vi "PulseHistogram.vi"() -> ()   [LabVIEW 2012]
doc: "This example demonstrates how to generate and acquire data up to eight channels using an NI 6587 adapter module. It generates either a constant value or a digital count-up pattern on the first eight even, odd, upper, or lower numbered channels of the DDC connector, and then acquires that pattern on the first eight odd, even, lower, or upper (respectively) numbered channels of the DDC connector. The data is generated on one cycle of the single-cycle timed loop and acquired on the next cycle of the loop. To properly verify the waveforms in this example, you must connect the first eight channels to the other eight channels on the DDC connector. For example, if you choose the Even to Odd Channel Configuration, connect the even numbered channels to the odd numbered channels (DIO 0 -> DIO 1, DIO 2 -> DIO 3,...DIO 14 -> DIO 15).\nThis getting started example is intended for lower clock rates depending on your setup. For high speed applications, refer to the Serdes Channel or Serdes Connector examples."
uses:
  <vilib>/Platform/TimedLoop/XDataNode/timing_clust.ctl
  <vilib>/Platform/TimedLoop/XDataNode/nitl_modes.ctl
  <vilib>/Platform/TimedLoop/XDataNode/wakeup.ctl
  <vilib>/rvi/Emulation/niFpgaSctlEmulationRegisterWithScheduler.vi
  <vilib>/rvi/eio/common/nirviEmuTemplateMethod_errors.vi
  <vilib>/rvi/Emulation/niFpgaSctlEmulationScheduler.vi
  <vilib>/rvi/FIFO/Fifo_Resource/nirvififoEmulationSetSize.vi
  <vilib>/rvi/DataTransferAndStorage/Container/Common/niFpgaContainerGetUniqueNameForEmu.vi
  <vilib>/rvi/Emulation/niFpgaSctlEmulationFifoFullMgr.vi
  <vilib>/rvi/errors/niFpgaSetErrorForExecOnDevCompSimple.vi
  <vilib>/rvi/eio/common/nirviEmuReportErrorAndStop.vi
  <vilib>/rvi/interface/RandomDataEmulation/nirviRandomDataFPGAFIFO.vi
  <vilib>/rvi/interface/RandomDataEmulation/niFpgaRandomDataHandleErrors.vi
  <vilib>/rvi/Emulation/niFpgaSctlEmulationResourceMgr.vi
  <vilib>/Platform/TimedLoop/XDataNode/XDataNode.xnode
  <vilib>/eio/EIONode/EIONode.xnode
  <vilib>/rvi/DataTransferAndStorage/Container/XNode/niFpgaContainer.xnode
  <vilib>/rvi/FIFO/Fifo_Resource/nirvififoEmulationClear.vi
  <vilib>/rvi/FIFO/Fifo_Resource/nirvififoEmulationRead.vi
  <vilib>/rvi/interface/RandomDataEmulation/nirviRandomDataFpgaReadWriteTemplate.vi
  <vilib>/rvi/FIFO/Fifo_Resource/nirvififoEmulationWrite.vi
  <vilib>/Platform/TimedLoop/XDataNode/XDNodeRunTimeDep.lvlib
panel:
  in  "Demultiplex":bool
  out "ToHostCh1A2FIFO overflow":bool
  out "ToHostCh1A1FIFO overflow":bool
  in  "Acquiring":bool
  in  "Acq_Reset":bool
  out "Interloop FIFO overflow":bool
  out "Onboard_Clock_Ready":bool
  in  "Onboard_Clock_Write_Data":u16
  in  "Onboard_Clock_Write":bool
  in  "Clock Source":u8(ring)=3 items=["Tristate"=0, "Sync Clock (PXIe only)"=2, "Adapter Module Onboard Clock"=3, "Strobe from Crosspoint Switch"=4, "Strobe Bypass"=5]
  in  "Xpoint_Switch_Write":bool
  out "Interloop FIFO timed out":bool
  out "ToHostLaserFIFO overflow":bool
  out "Xpoint_Switch_Ready":bool
  in  "Commit":bool
  # "PulseHistogram"
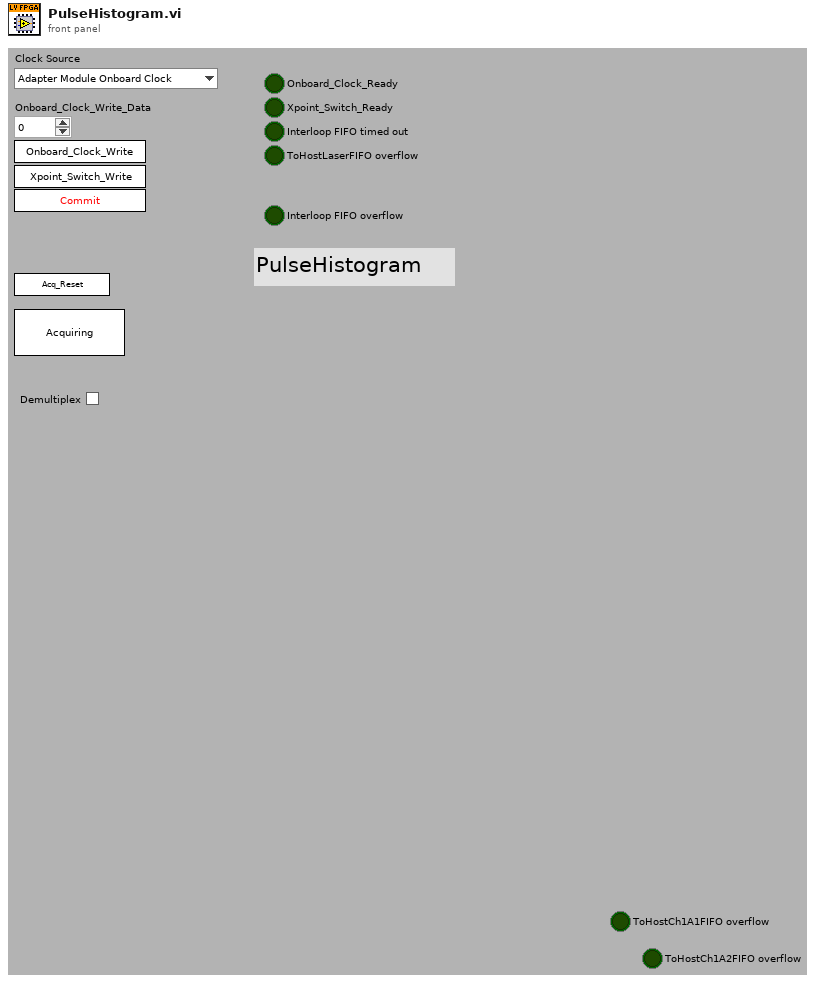
[diagram p1: front panel]
types:
  T1 = typedef "XDNodeRunTimeDep.lvlib/timing_clust.ctl" = cluster{"Expected End [f-1]":u64, "Actual End [f-1]":u64, "Finished Late? [f-1]":bool, "Expected End [i-1]":u64, "Actual End [i-1]":u64, "Finished Late? [i-1]":bool, "Expected Start [i]":u64, "Actual Start [i]":u64, "Expected Start [f]":u64, "Actual Start [f]":u64, "Source Name":string, "Structure Name":string, "Period":i64, "Deadline":i64, "Offset":i64, "Start":i64, "Priority":i32, "Timeout":i32, "Mode":T2, "Wakeup Reason":T3, "Error":errorcluster, "Source Type":string, "Secondary Source Type":string, "Global End Time":u64, "Global Start Time":u64, "Frame Duration":u64, "Iteration Duration":u64, "Assigned CPU":i32, "I/O Scan Engine Mode":u32}
  T2 = typedef "XDNodeRunTimeDep.lvlib/nitl_modes.ctl" = enum32{"No Change", "Process missed periods, maintain original phase", "Discard missed periods, maintain original phase", "Process missed periods, ignore original phase", "Discard missed periods, ignore original phase"}
  T3 = typedef "XDNodeRunTimeDep.lvlib/wakeup.ctl" = enum32{"Normal", "Aborted", "Asynchronous wakeup", "Timing source error", "Timed loop error", "Timeout"}
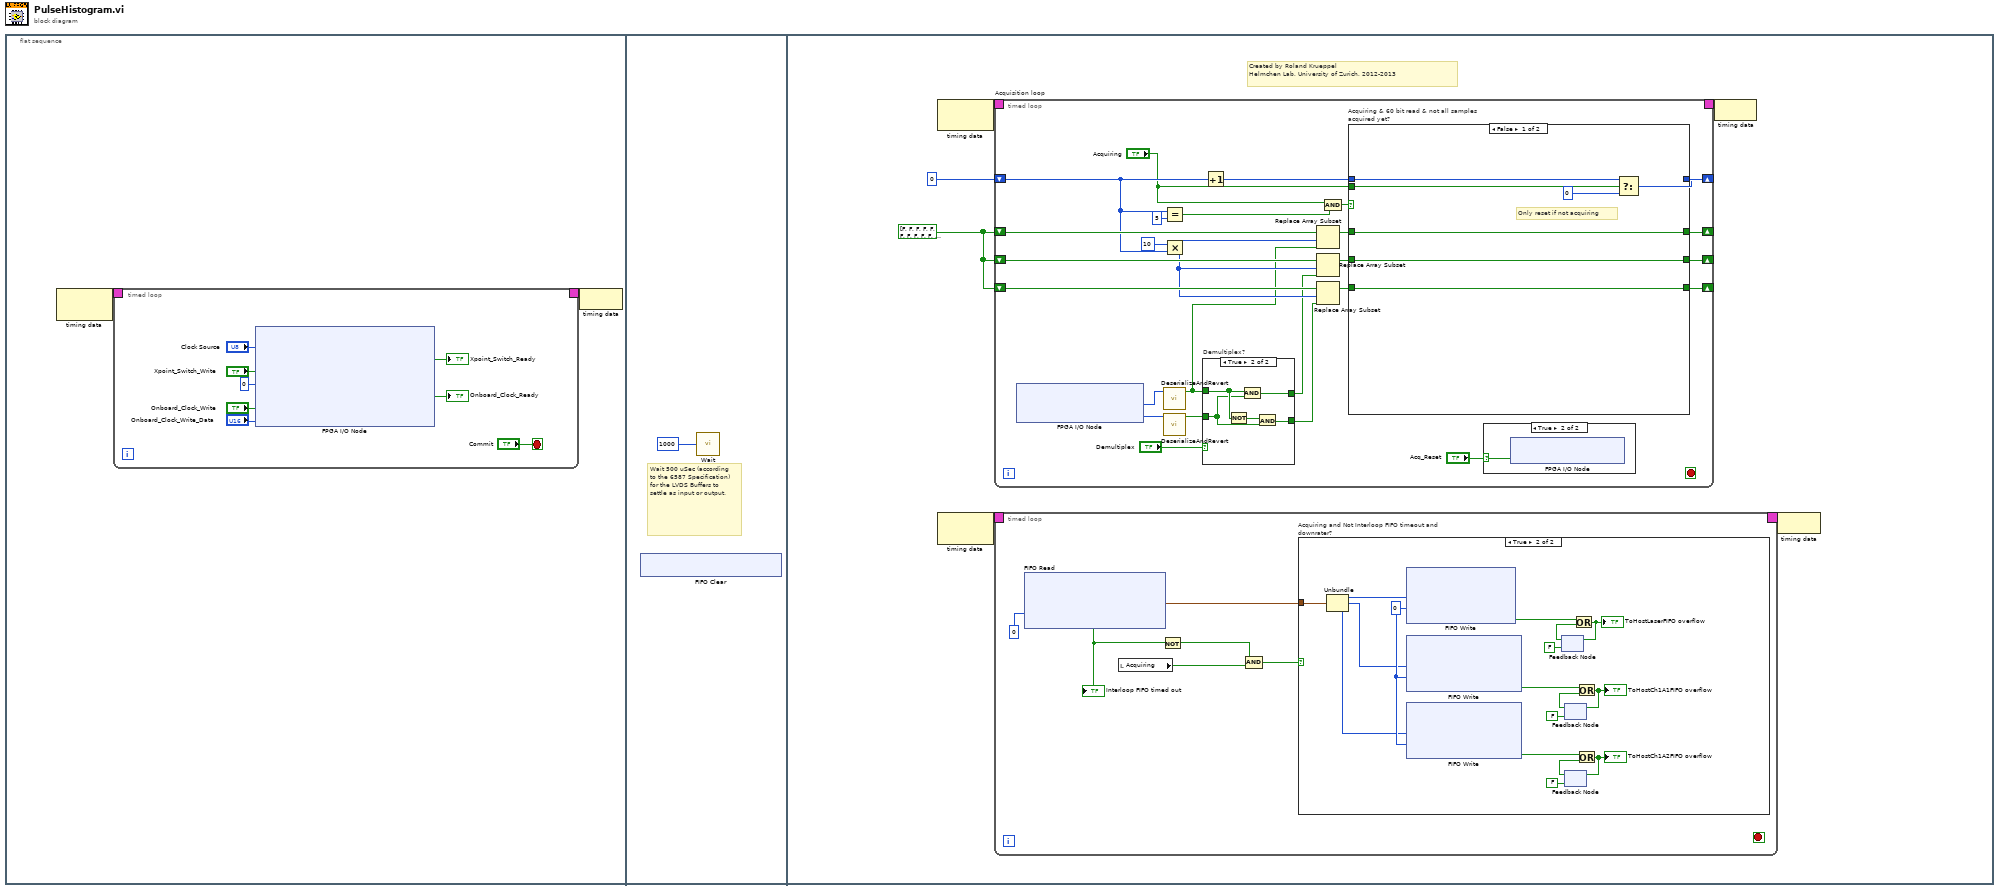
[diagram p0: block diagram]
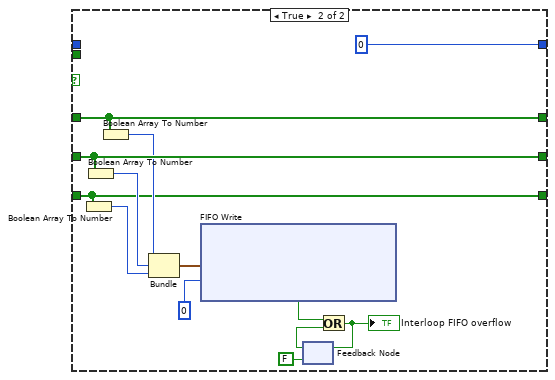
[diagram p4: hidden frame]
diagram:
  n1 = flat-sequence {
    frame #0 {
      n2 = node-c288() -> (w2:T1)  [unwired: 1 in]
      n3 = timed-loop {
        timing: w2 -> [_]
        timing-out: [_] -> w1
        stop <- "Commit" stop-if-true
        n4 = xnode "FPGA I/O Node"("IO Module\\Acq_IO_Clock_Source"="Clock Source", "IO Module\\Xpoint_Switch_Write"="Xpoint_Switch_Write", "IO Module\\LVDS_Data_Dir"=u16 0 ("IO Module\\LVDS_Data_Dir"), "IO Module\\Onboard_Clock_Write"="Onboard_Clock_Write", "IO Module\\Onboard_Clock_Write_Data"="Onboard_Clock_Write_Data") -> ("IO Module\\Xpoint_Switch_Ready"=→"Xpoint_Switch_Ready":bool, "IO Module\\Onboard_Clock_Ready"=→"Onboard_Clock_Ready":bool)  [unwired: 7 in, 7 out]
      }
      n5 = node-c288(w1) -> ()
    }
    frame #1 {
      # "Wait 500 uSec (according to the 6587 Specification) for the LVDS Buffers to settle as input or output."
      n6 = xnode ("FIFO Clear")() -> ()  [unwired: 1 in, 1 out]
      n7 = call "Wait"("Count(uSec)"=u32 1000 ("Wait (uSec)")) -> ()  [unwired: 1 out]
    }
    frame #2 {
      w16 = bool[] [FALSE, FALSE, FALSE, FALSE, FALSE, FALSE, FALSE, FALSE, FALSE, FALSE, FALSE, FALSE, FALSE, FALSE, FALSE, FALSE, FALSE, FALSE, FALSE, FALSE, FALSE, FALSE, FALSE, FALSE, FALSE, FALSE, FALSE, FALSE, FALSE, FALSE, FALSE, FALSE, FALSE, FALSE, FALSE, FALSE, FALSE, FALSE, FALSE, FALSE, FALSE, FALSE, FALSE, FALSE, FALSE, FALSE, FALSE, FALSE, FALSE, FALSE, FALSE, FALSE, FALSE, FALSE, FALSE, FALSE, FALSE, FALSE, FALSE, FALSE, FALSE, FALSE, FALSE, FALSE] ("Boolean array")
      # "Created by Roland Krueppel\nHelmchen Lab, University of Zurich, 2012-2013"
      n8 = node-c288() -> (w19:T1)  [unwired: 1 in]
      n9 = node-c288() -> (w21:T1)  [unwired: 1 in]
      n10 = timed-loop "Acquisition loop" {
        timing: w19 -> [_]
        timing-out: [_] -> w18
        shift-right: [w39] -> _
        shift-left: w16 -> [w47]
        shift-right: [w38] -> _
        shift-left: w16 -> [w46]
        shift-right: [w37] -> _
        shift-left: 0 -> [w36]
        shift-right: [w27] -> _
        shift-left: w16 -> [w30]
        stop <- _ stop-if-true
        n11 = xnode "FPGA I/O Node"() -> ("IO Module\\LVDS_Ch0_Rd"=w34:u16, "IO Module\\LVDS_Ch1_Rd"=w33:u16)  [unwired: 2 in, 2 out]
        n12 = Equal?(x=w36, y=5) -> (x = y?=w43:bool)
        n13 = Multiply(x=10 ("y"), y=w36) -> (x*y=w29:i32)
        n14 = call "DeserializeAndRevert.vi"("U16 input"=w34) -> ("10bit output"=w25:bool[])  [unwired: 10 in]
        n15 = call "DeserializeAndRevert.vi"("U16 input"=w33) -> ("10bit output"=w24:bool[])  [unwired: 10 in]
        n16 = case "Demultiplex?" shown="True" "Demultiplex" {
          tunnel: [w48 w53] -> w26
          tunnel: w25 -> [_ w52]
          tunnel: w24 -> [w48 w50]
          tunnel: [w48 w49] -> w23
          frame False {
          }
          frame True {
            n17 = Not(x=w52) -> (.not. x?=w51:bool[])
            n18 = And(x=w52, y=w50) -> (x .and. y?=w53:bool[])
            n19 = And(x=w51, y=w50) -> (x .and. y?=w49:bool[])
          }
        }
        n20 = Increment(x=w36) -> (x+1=w35:i32)
        n21 = Replace Array Subset(array=w47, new element=w25, index=w29) -> (w41:bool[])
        n22 = Replace Array Subset(array=w46, new element=w26, index=w29) -> (w40:bool[])
        n23 = Replace Array Subset(array=w30, new element=w23, index=w29) -> (w28:bool[])
        n24 = Compound Arithmetic op=AND("Acquiring", w43) -> (w42:bool)
        n25 = case "Acquiring & 60 bit read & not all samples acquired yet?" shown="False" w42 {
          tunnel: w41 -> [w61 w72]
          tunnel: w40 -> [w60 w73]
          tunnel: [w61 w72] -> w39
          tunnel: [w60 w73] -> w38
          tunnel: [w58 0] -> w37
          tunnel: w35 -> [w59 _]
          tunnel: "Acquiring" -> [w56 _]
          tunnel: w28 -> [w55 w62]
          tunnel: [w55 w62] -> w27
          frame False {
            # "Only reset if not acquiring"
            n26 = Select(t=w59, s=w56, f=0) -> (s? t:f=w58:i32)
          }
          frame True {
            n27 = Boolean Array To Number(Boolean array=w62) -> (number=w63:u64)
            n28 = Boolean Array To Number(Boolean array=w73) -> (number=w64:u64)
            n29 = Boolean Array To Number(Boolean array=w72) -> (number=w65:u64)
            n30 = Bundle(w65, w64, w63) -> (w66:cluster{u64, u64, u64})  [unwired: 1 in]
            n31 = xnode ("FIFO Write")("Element"=w66, "Timeout"=0) -> ("Timed Out?"=w70:bool)  [unwired: 1 in, 1 out]
            n32 = feedback #1(FALSE) -> (w68:bool)
            n33 = Or(x=w70, y=w68) -> (x .or. y?=w69:bool)
            "Interloop FIFO overflow" <- w69
            n34 = feedback-in #1(w69) -> ()
          }
        }
        n35 = case shown="True" "Acq_Reset" {
          selector: "Acq_Reset" -> [_ w54]
          frame False {
          }
          frame True {
            n36 = xnode "FPGA I/O Node"("IO Module\\Acq_Reset"=w54) -> ()  [unwired: 1 in, 1 out]
          }
        }
      }
      n37 = timed-loop {
        timing: w21 -> [_]
        timing-out: [_] -> w20
        stop <- _ stop-if-true
        n38 = xnode ("FIFO Read")("Timeout"=0) -> ("Element"=w83:cluster{"Laser":u64, "Ch1 A1":u64, "Ch1 A2":u64}, "Timed Out?"=w80:bool)  [unwired: 1 in, 1 out]
        "Interloop FIFO timed out" <- w80
        n39 = local read "Acquiring"() -> (w82:bool)
        n40 = Not(x=w80) -> (.not. x?=w81:bool)
        n41 = Compound Arithmetic op=AND(w81, w82) -> (w79:bool)
        n42 = case "Acquiring and Not Interloop FIFO timeout and downrater?" shown="True" w79 {
          tunnel: w83 -> [_ w101]
          frame False {
          }
          frame True {
            w87 = 0 ("Timeout")
            n43 = Unbundle(w101) -> ("Laser"=w96:u64, "Ch1 A1"=w86:u64, "Ch1 A2"=w85:u64)
            n44 = xnode ("FIFO Write")("Element"=w96, "Timeout"=w87) -> ("Timed Out?"=w97:bool)  [unwired: 1 in, 1 out]
            n45 = xnode ("FIFO Write")("Element"=w86, "Timeout"=w87) -> ("Timed Out?"=w92:bool)  [unwired: 1 in, 1 out]
            n46 = xnode ("FIFO Write")("Element"=w85, "Timeout"=w87) -> ("Timed Out?"=w88:bool)  [unwired: 1 in, 1 out]
            n47 = feedback #2(FALSE) -> (w100:bool)
            n48 = feedback #3(FALSE) -> (w95:bool)
            n49 = feedback #4(FALSE) -> (w91:bool)
            n50 = Or(x=w97, y=w100) -> (x .or. y?=w98:bool)
            "ToHostLaserFIFO overflow" <- w98
            n51 = feedback-in #2(w98) -> ()
            n52 = Or(x=w92, y=w95) -> (x .or. y?=w93:bool)
            "ToHostCh1A1FIFO overflow" <- w93
            n53 = feedback-in #3(w93) -> ()
            n54 = Or(x=w88, y=w91) -> (x .or. y?=w89:bool)
            "ToHostCh1A2FIFO overflow" <- w89
            n55 = feedback-in #4(w89) -> ()
          }
        }
      }
      n56 = node-c288(w18) -> ()
      n57 = node-c288(w20) -> ()
    }
  }
